vi "Close.mono.vi"(11 "Mono":T1) -> ()   [LabVIEW 2022 SP3]
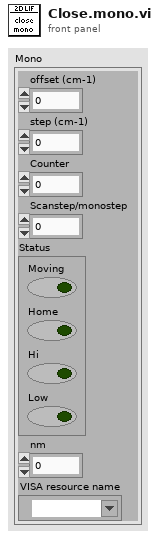
[diagram p1: front panel]
types:
  T1 = cluster{"offset (cm-1)":dbl, "step (cm-1)":dbl, "Counter":dbl, "Scanstep/monostep":i32, "Status":cluster{"Moving":bool, "Home":bool, "Hi":bool, "Low":bool}, "nm":dbl, "VISA resource name":refnum<visa-resource-name>}
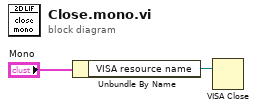
[diagram p0: block diagram]
diagram:
  n1 = Unbundle By Name("Mono") -> ("VISA resource name"=w1:refnum<visa-resource-name>)
  n2 = VISA Close(VISA resource name=w1) -> ()  [unwired: 1 in, 1 out]
